vi "SentinelController v35 good v11.vi"() -> ()   [LabVIEW 2011] (continued)
                                n1651 = local read "tester tt start hid"() -> (w1552:u32)
                                n1652 = local read "tester tt end hid"() -> (w1553:u32)
                                n1653 = Subtract(x=w1553, y=w1552) -> (x-y=w1551:u32)
                                n1654 = Divide(x=w1551, y=u32 1000) -> (x/y=w1549:dbl)
                                n1655 = local write "SC measured test time hid"(w1549) -> ()
                                }
                                frame #3 {
                                n1656 = local read "H1 Lock"() -> (w1554:bool)
                                n1657 = case shown="False" w1554 {
                                frame False {
                                n1658 = local read "H2 Lock"() -> (w1555:bool)
                                n1659 = case shown="False" w1555 {
                                frame False {
                                n1660 = One Button Dialog(message="Fatal error 202:\nThe SC responded to a handler being ready with devices\nto test, but when the SC received binning data, no handler had a lock. \nPlease report this bug to Celerint at www.celerint.com  ") -> ()  [unwired: 1 in, 1 out]
                                }
                                frame True {
                                n1661 = local read "H2 online"() -> (w1576:bool)
                                n1662 = local read "Tandem\nfloorspace area"() -> (w1559:i32)
                                n1663 = local read "Std cell \nfloorspace area"() -> (w1587:i32)
                                n1664 = case shown="True" w1576 {
                                tunnel: [0 w1591] -> w1577
                                frame False {
                                }
                                frame True {
                                n1665 = local read "H2 UPH"() -> (w1592:cluster{u32, u32})
                                n1666 = Unbundle(w1592) -> (w1591:u32)  [unwired: 1 out]
                                }
                                }
                                n1667 = local read "System UPH"() -> (w1558:u32)
                                n1668 = local read "UPH"() -> (w1588:dbl)
                                n1669 = Divide(x=w1558, y=w1559) -> (x/y=w1557:dbl)
                                n1670 = local write "Tandem UPH\nper unit area"(w1557) -> ()
                                n1671 = Divide(x=w1588, y=w1587) -> (x/y=w1589:dbl)
                                n1672 = local read "Std hourly\ncost ($/hr)"() -> (w1584:dbl)
                                n1673 = local read "H1 UPH"() -> (w1586:cluster{u32, u32})
                                n1674 = local write "H1 UPH per unit area"(w1589) -> ()
                                n1675 = local read "Utilization (%)"() -> (w1569:u32)
                                n1676 = local read "Tandem hourly\ncost ($/hr)"() -> (w1585:dbl)
                                n1677 = local read "# of devices to test"() -> (w1575:u32)
                                n1678 = Unbundle(w1586) -> (w1578:u32)  [unwired: 1 out]
                                n1679 = local read "Hours per month"() -> (w1570:i32)
                                n1680 = local write "Calc H2 UPH"(w1577) -> ()
                                n1681 = local write "Calc H1 UPH"(w1578) -> ()
                                n1682 = local read "UPH"() -> (w1583:dbl)
                                n1683 = Add(x=w1578, y=w1577) -> (x+y=w1565:u32)
                                n1684 = Divide(x=w1569, y=u32 100) -> (x/y=w1568:dbl)
                                n1685 = Divide(x=w1575, y=w1565) -> (x/y=w1574:dbl)
                                n1686 = Multiply(x=w1570, y=w1568) -> (x*y=w1566:dbl)
                                n1687 = Divide(x=w1584, y=w1583) -> (x/y=w1582:dbl)
                                n1688 = Divide(x=w1585, y=w1565) -> (x/y=w1580:dbl)
                                n1689 = local write "System UPH"(w1565) -> ()
                                n1690 = local write "Calc\nsystem UPH"(w1565) -> ()
                                n1691 = local read "# of devices to test"() -> (w1563:u32)
                                n1692 = Divide(x=w1574, y=w1566) -> (x/y=w1573:dbl)
                                n1693 = Multiply(x=w1582, y=100.0) -> (x*y=w1561:dbl)
                                n1694 = Multiply(x=w1580, y=100.0) -> (x*y=w1560:dbl)
                                n1695 = local write "Std unit cost\n(cents/device)"(w1561) -> ()
                                n1696 = local write "Tandem unit cost\n(cents/device)"(w1560) -> ()
                                n1697 = Subtract(x=w1561, y=w1560) -> (x-y=w1564:dbl)
                                n1698 = Multiply(x=w1573, y=30) -> (x*y=w1571:dbl)
                                n1699 = Multiply(x=w1563, y=w1564) -> (x*y=w1562:dbl)
                                n1700 = local write "Calendar days required\nfor testing all units"(w1571) -> ()
                                n1701 = local write "$ saved"(w1562) -> ()
                                }
                                }
                                }
                                frame True {
                                n1702 = local read "H1 online"() -> (w1613:bool)
                                n1703 = local read "Tandem\nfloorspace area"() -> (w1625:i32)
                                n1704 = local read "Std cell \nfloorspace area"() -> (w1618:i32)
                                n1705 = case shown="True" w1613 {
                                tunnel: [0 w1627] -> w1593
                                frame False {
                                }
                                frame True {
                                n1706 = local read "H1 UPH"() -> (w1628:cluster{u32, u32})
                                n1707 = Unbundle(w1628) -> (w1627:u32)  [unwired: 1 out]
                                }
                                }
                                n1708 = local read "System UPH"() -> (w1624:u32)
                                n1709 = local read "H2 calc UPH"() -> (w1619:dbl)
                                n1710 = Divide(x=w1624, y=w1625) -> (x/y=w1596:dbl)
                                n1711 = Divide(x=w1619, y=w1618) -> (x/y=w1597:dbl)
                                n1712 = local write "Tandem UPH\nper unit area"(w1596) -> ()
                                n1713 = local write "H2 UPH per unit area"(w1597) -> ()
                                n1714 = local read "Std hourly\ncost ($/hr)"() -> (w1621:dbl)
                                n1715 = local read "H2 UPH"() -> (w1623:cluster{u32, u32})
                                n1716 = local read "Utilization (%)"() -> (w1603:u32)
                                n1717 = local read "Tandem hourly\ncost ($/hr)"() -> (w1622:dbl)
                                n1718 = local read "# of devices to test"() -> (w1609:u32)
                                n1719 = local read "Hours per month"() -> (w1604:i32)
                                n1720 = Unbundle(w1623) -> (w1599:u32)  [unwired: 1 out]
                                n1721 = local write "Calc H1 UPH"(w1593) -> ()
                                n1722 = local write "Calc H2 UPH"(w1599) -> ()
                                n1723 = local read "UPH"() -> (w1620:dbl)
                                n1724 = Add(x=w1593, y=w1599) -> (x+y=w1598:u32)
                                n1725 = Divide(x=w1603, y=u32 100) -> (x/y=w1602:dbl)
                                n1726 = local write "System UPH"(w1598) -> ()
                                n1727 = local write "Calc\nsystem UPH"(w1598) -> ()
                                n1728 = Divide(x=w1609, y=w1598) -> (x/y=w1608:dbl)
                                n1729 = Multiply(x=w1604, y=w1602) -> (x*y=w1600:dbl)
                                n1730 = Divide(x=w1621, y=w1620) -> (x/y=w1617:dbl)
                                n1731 = Divide(x=w1622, y=w1598) -> (x/y=w1615:dbl)
                                n1732 = local read "# of devices to test"() -> (w1611:u32)
                                n1733 = Divide(x=w1608, y=w1600) -> (x/y=w1607:dbl)
                                n1734 = Multiply(x=w1617, y=100.0) -> (x*y=w1595:dbl)
                                n1735 = Multiply(x=w1615, y=100.0) -> (x*y=w1594:dbl)
                                n1736 = local write "Std unit cost\n(cents/device)"(w1595) -> ()
                                n1737 = local write "Tandem unit cost\n(cents/device)"(w1594) -> ()
                                n1738 = Subtract(x=w1595, y=w1594) -> (x-y=w1612:dbl)
                                n1739 = Multiply(x=w1607, y=30) -> (x*y=w1605:dbl)
                                n1740 = Multiply(x=w1611, y=w1612) -> (x*y=w1610:dbl)
                                n1741 = local write "Calendar days required\nfor testing all units"(w1605) -> ()
                                n1742 = local write "$ saved"(w1610) -> ()
                                }
                                }
                                }
                                frame #4 {
                                # "when this loop unlocks the handlers,\nthe handler interface loops are free to continue\nto send the binning information to their\nrespective handlers.  Each handler interface \nloop using the \"binning string hidden\" to do\nthis.  That is why, here, there is no writing of\nthe binning informatrion to a handler.  \nThat is done in the handler interface loops."
                                n1743 = local write "H1 Lock"(FALSE ("H1 Lock")) -> ()
                                n1744 = local write "H2 Lock"(FALSE ("H1 Lock")) -> ()
                                }
                                frame #5 {
                                n1745 = local read "Tester online"() -> (w1631:bool)
                                n1746 = local read "POWER"() -> (w1633:bool)
                                n1747 = Compound Arithmetic op=AND(w1631, w1633) -> (w1632:bool)
                                n1748 = case shown="True" w1632 {
                                frame False {
                                n1749 = local write "SC handler states hid"(SC_handler_states."closing bus" ("SC virtual handler states")) -> ()
                                }
                                frame True {
                                n1750 = local write "SC handler states hid"(SC_handler_states."waiting on event" ("SC virtual handler states")) -> ()
                                }
                                }
                                }
                                }
                              }
                              frame "responding to BINON" {
                                n1751 = local read "Last locked handler hid"() -> (w1638:enum16{"H1", "H2"})
                                n1752 = Equal?(x=w1638, y=enum16{"H1", "H2"}."H1") -> (x = y?=w1636:bool)
                                n1753 = case shown="True" w1636 {
                                frame False {
                                n1754 = local read "Last locked handler hid"() -> (w1642:enum16{"H1", "H2"})
                                n1755 = Equal?(x=w1642, y=enum16{"H1", "H2"}."H2") -> (x = y?=w1641:bool)
                                n1756 = case shown="True" w1641 {
                                frame False {
                                }
                                frame True {
                                n1757 = flat-sequence {
                                frame #0 {
                                n1758 = while {
                                stop <- w1646 stop-if-true
                                n1759 = local read "H2 echo hid"() -> (w1644:string)
                                n1760 = String Length(string=w1644) -> (length=w1647:i32)
                                n1761 = Greater Than 0?(x=w1647) -> (x > 0?=w1646:bool)
                                n1762 = Wait (ms)(milliseconds to wait=u32 1) -> ()  [unwired: 1 out]
                                }
                                }
                                frame #1 {
                                # "4"
                                n1763 = local read "GPIB Bus 0 traffic"() -> (w1654:string)
                                n1764 = local read "H2 echo hid"() -> (w1648:string)
                                n1765 = local read "VISA bus 0 resource name out hid"() -> (w1658:refnum<visa-resource-name>)
                                n1766 = local read "VISA bus 0 error out hid"() -> (w1657:errorcluster)
                                n1767 = call <vilib>:"Trim Whitespace.vi"("string"=w1648) -> ("trimmed string"=w1649:string)  [unwired: 1 in]
                                n1768 = VISA Write(VISA resource name=w1658, write buffer=w1648, error in (no error)=w1657) -> (VISA resource name out=w1656:refnum<visa-resource-name>, error out=w1655:errorcluster)  [unwired: 1 out]
                                n1769 = Concatenate Strings(w1654, "\r\n", "Bus 0 write: " ("string"), w1649) -> (w1652:string)
                                n1770 = local write "VISA bus 0 resource name out hid"(w1656) -> ()
                                n1771 = Unbundle By Name(w1655) -> ("status"=w1650:bool)
                                n1772 = local write "VISA bus 0 error out hid"(w1655) -> ()
                                n1773 = local write "GPIB Bus 0 traffic"(w1652) -> ()
                                n1774 = local write "GPIB bus 0 write error"(w1650) -> ()
                                }
                                frame #2 {
                                n1775 = local write "SC handler states hid"(SC_handler_states."waiting on event" ("SC Test Interface States")) -> ()
                                }
                                }
                                }
                                }
                                }
                                frame True {
                                n1776 = flat-sequence {
                                frame #0 {
                                n1777 = while {
                                i -> [w1660]
                                stop <- w1662 stop-if-true
                                n1778 = local read "H1 echo hid"() -> (w1664:string)
                                n1779 = String Length(string=w1664) -> (length=w1663:i32)
                                n1780 = Greater Than 0?(x=w1663) -> (x > 0?=w1662:bool)
                                n1781 = Wait (ms)(milliseconds to wait=u32 1) -> ()  [unwired: 1 out]
                                "Numeric 4" <- w1660
                                }
                                }
                                frame #1 {
                                n1782 = local read "GPIB Bus 0 traffic"() -> (w1671:string)
                                n1783 = local read "VISA bus 0 resource name out hid"() -> (w1675:refnum<visa-resource-name>)
                                n1784 = local read "H1 echo hid"() -> (w1665:string)
                                n1785 = local read "VISA bus 0 error out hid"() -> (w1674:errorcluster)
                                n1786 = VISA Write(VISA resource name=w1675, write buffer=w1665, error in (no error)=w1674) -> (VISA resource name out=w1673:refnum<visa-resource-name>, error out=w1672:errorcluster)  [unwired: 1 out]
                                n1787 = call <vilib>:"Trim Whitespace.vi"("string"=w1665) -> ("trimmed string"=w1666:string)  [unwired: 1 in]
                                n1788 = local write "VISA bus 0 resource name out hid"(w1673) -> ()
                                n1789 = Unbundle By Name(w1672) -> ("status"=w1667:bool)
                                n1790 = local write "VISA bus 0 error out hid"(w1672) -> ()
                                n1791 = Concatenate Strings(w1671, "\r\n", "Bus 0 write: " ("string"), w1666) -> (w1669:string)
                                n1792 = local write "GPIB bus 0 write error"(w1667) -> ()
                                n1793 = local write "GPIB Bus 0 traffic"(w1669) -> ()
                                }
                                frame #2 {
                                n1794 = local write "SC handler states hid"(SC_handler_states."waiting on event" ("SC Test Interface States")) -> ()
                                }
                                }
                                }
                                }
                              }
                              frame "ECHONG" {
                                n1795 = flat-sequence {
                                frame #0 {
                                # "Echo was returned to the tester via the BINON state"
                                n1796 = local read "H1 Lock"() -> (w1679:bool)
                                n1797 = case shown="True" w1679 {
                                frame False {
                                n1798 = local read "H2 Lock"() -> (w1680:bool)
                                n1799 = case shown="True" w1680 {
                                frame False {
                                }
                                frame True {
                                n1800 = local read "GPIB Bus 0 traffic"() -> (w1684:string)
                                n1801 = Concatenate Strings(w1684, "\r\n", "Bus 0: ECHONG received for H2. Retrying." ("string")) -> (w1682:string)
                                n1802 = local write "GPIB Bus 0 traffic"(w1682) -> ()
                                }
                                }
                                }
                                frame True {
                                n1803 = local read "GPIB Bus 0 traffic"() -> (w1688:string)
                                n1804 = Concatenate Strings(w1688, "\r\n", "Bus 0: ECHONG received for H1. Retrying." ("string")) -> (w1686:string)
                                n1805 = local write "GPIB Bus 0 traffic"(w1686) -> ()
                                }
                                }
                                }
                                frame #1 {
                                n1806 = local write "SC handler states hid"(SC_handler_states."waiting on event" ("SC Test Interface States")) -> ()
                                }
                                }
                              }
                              frame "ECHOOK" {
                                n1807 = flat-sequence {
                                frame #0 {
                                # "Echo was returned to the tester via the BINON state"
                                n1808 = local read "Last locked handler hid"() -> (w1694:enum16{"H1", "H2"})
                                n1809 = Equal?(x=w1694, y=enum16{"H1", "H2"}."H1") -> (x = y?=w1692:bool)
                                n1810 = case shown="True" w1692 {
                                frame False {
                                n1811 = local read "Last locked handler hid"() -> (w1696:enum16{"H1", "H2"})
                                n1812 = Equal?(x=w1696, y=enum16{"H1", "H2"}."H2") -> (x = y?=w1695:bool)
                                n1813 = case shown="True" w1695 {
                                frame False {
                                }
                                frame True {
                                n1814 = local read "GPIB Bus 0 traffic"() -> (w1701:string)
                                n1815 = Concatenate Strings(w1701, "\r\n", "Bus 0: ECHOOK received for H2." ("string")) -> (w1699:string)
                                n1816 = local write "GPIB Bus 0 traffic"(w1699) -> ()
                                }
                                }
                                }
                                frame True {
                                n1817 = local read "GPIB Bus 0 traffic"() -> (w1705:string)
                                n1818 = Concatenate Strings(w1705, "\r\n", "Bus 0: ECHOOK received for H1." ("string")) -> (w1703:string)
                                n1819 = local write "GPIB Bus 0 traffic"(w1703) -> ()
                                }
                                }
                                }
                                frame #1 {
                                n1820 = Tick Count (ms)() -> (millisecond timer value=w1706:u32)
                                n1821 = Tick Count (ms)() -> (millisecond timer value=w1707:u32)
                                n1822 = local write "tester wt start hid"(w1706) -> ()
                                n1823 = local write "tester tt end hid"(w1707) -> ()
                                }
                                frame #2 {
                                n1824 = local read "tester tt start hid"() -> (w1711:u32)
                                n1825 = local read "tester tt end hid"() -> (w1712:u32)
                                n1826 = Subtract(x=w1712, y=w1711) -> (x-y=w1710:u32)
                                n1827 = Divide(x=w1710, y=u32 1000) -> (x/y=w1708:dbl)
                                n1828 = local write "SC measured test time hid"(w1708) -> ()
                                }
                                frame #3 {
                                n1829 = local read "Last locked handler hid"() -> (w1713:enum16{"H1", "H2"})
                                n1830 = case shown="\"H1\", Default" w1713 {
                                frame "H1", Default {
                                n1831 = local read "H1 online"() -> (w1734:bool)
                                n1832 = local read "Tandem\nfloorspace area"() -> (w1746:i32)
                                n1833 = local read "Std cell \nfloorspace area"() -> (w1739:i32)
                                n1834 = case shown="True" w1734 {
                                tunnel: [0 w1748] -> w1714
                                frame False {
                                }
                                frame True {
                                n1835 = local read "H1 UPH"() -> (w1749:cluster{u32, u32})
                                n1836 = Unbundle(w1749) -> (w1748:u32)  [unwired: 1 out]
                                }
                                }
                                n1837 = local read "System UPH"() -> (w1745:u32)
                                n1838 = local read "H2 calc UPH"() -> (w1740:dbl)
                                n1839 = Divide(x=w1745, y=w1746) -> (x/y=w1717:dbl)
                                n1840 = Divide(x=w1740, y=w1739) -> (x/y=w1718:dbl)
                                n1841 = local write "Tandem UPH\nper unit area"(w1717) -> ()
                                n1842 = local write "H2 UPH per unit area"(w1718) -> ()
                                n1843 = local read "Std hourly\ncost ($/hr)"() -> (w1742:dbl)
                                n1844 = local read "H2 UPH"() -> (w1744:cluster{u32, u32})
                                n1845 = local read "Utilization (%)"() -> (w1724:u32)
                                n1846 = local read "Tandem hourly\ncost ($/hr)"() -> (w1743:dbl)
                                n1847 = local read "# of devices to test"() -> (w1730:u32)
                                n1848 = local read "Hours per month"() -> (w1725:i32)
                                n1849 = Unbundle(w1744) -> (w1720:u32)  [unwired: 1 out]
                                n1850 = local write "Calc H1 UPH"(w1714) -> ()
                                n1851 = local write "Calc H2 UPH"(w1720) -> ()
                                n1852 = local read "UPH"() -> (w1741:dbl)
                                n1853 = Add(x=w1714, y=w1720) -> (x+y=w1719:u32)
                                n1854 = Divide(x=w1724, y=u32 100) -> (x/y=w1723:dbl)
                                n1855 = Divide(x=w1742, y=w1741) -> (x/y=w1738:dbl)
                                n1856 = Divide(x=w1743, y=w1719) -> (x/y=w1736:dbl)
                                n1857 = Divide(x=w1730, y=w1719) -> (x/y=w1729:dbl)
                                n1858 = Multiply(x=w1725, y=w1723) -> (x*y=w1721:dbl)
                                n1859 = local write "System UPH"(w1719) -> ()
                                n1860 = local write "Calc\nsystem UPH"(w1719) -> ()
                                n1861 = local read "# of devices to test"() -> (w1732:u32)
                                n1862 = Divide(x=w1729, y=w1721) -> (x/y=w1728:dbl)
                                n1863 = Multiply(x=w1738, y=100.0) -> (x*y=w1716:dbl)
                                n1864 = Multiply(x=w1736, y=100.0) -> (x*y=w1715:dbl)
                                n1865 = local write "Tandem unit cost\n(cents/device)"(w1715) -> ()
                                n1866 = local write "Std unit cost\n(cents/device)"(w1716) -> ()
                                n1867 = Subtract(x=w1716, y=w1715) -> (x-y=w1733:dbl)
                                n1868 = Multiply(x=w1728, y=30) -> (x*y=w1726:dbl)
                                n1869 = Multiply(x=w1732, y=w1733) -> (x*y=w1731:dbl)
                                n1870 = local write "Calendar days required\nfor testing all units"(w1726) -> ()
                                n1871 = local write "$ saved"(w1731) -> ()
                                }
                                frame "H2" {
                                n1872 = local read "H2 online"() -> (w1769:bool)
                                n1873 = local read "Tandem\nfloorspace area"() -> (w1752:i32)
                                n1874 = local read "Std cell \nfloorspace area"() -> (w1780:i32)
                                n1875 = case shown="True" w1769 {
                                tunnel: [0 w1784] -> w1770
                                frame False {
                                }
                                frame True {
                                n1876 = local read "H2 UPH"() -> (w1785:cluster{u32, u32})
                                n1877 = Unbundle(w1785) -> (w1784:u32)  [unwired: 1 out]
                                }
                                }
                                n1878 = local read "System UPH"() -> (w1751:u32)
                                n1879 = local read "UPH"() -> (w1781:dbl)
                                n1880 = Divide(x=w1751, y=w1752) -> (x/y=w1750:dbl)
                                n1881 = local write "Tandem UPH\nper unit area"(w1750) -> ()
                                n1882 = Divide(x=w1781, y=w1780) -> (x/y=w1782:dbl)
                                n1883 = local read "Std hourly\ncost ($/hr)"() -> (w1777:dbl)
                                n1884 = local read "H1 UPH"() -> (w1779:cluster{u32, u32})
                                n1885 = local read "Utilization (%)"() -> (w1762:u32)
                                n1886 = local write "H1 UPH per unit area"(w1782) -> ()
                                n1887 = local read "Tandem hourly\ncost ($/hr)"() -> (w1778:dbl)
                                n1888 = local read "# of devices to test"() -> (w1768:u32)
                                n1889 = Unbundle(w1779) -> (w1771:u32)  [unwired: 1 out]
                                n1890 = local read "Hours per month"() -> (w1763:i32)
                                n1891 = local write "Calc H1 UPH"(w1771) -> ()
                                n1892 = local write "Calc H2 UPH"(w1770) -> ()
                                n1893 = local read "UPH"() -> (w1776:dbl)
                                n1894 = Add(x=w1771, y=w1770) -> (x+y=w1758:u32)
                                n1895 = Divide(x=w1762, y=u32 100) -> (x/y=w1761:dbl)
                                n1896 = Divide(x=w1777, y=w1776) -> (x/y=w1775:dbl)
                                n1897 = Divide(x=w1778, y=w1758) -> (x/y=w1773:dbl)
                                n1898 = Divide(x=w1768, y=w1758) -> (x/y=w1767:dbl)
                                n1899 = Multiply(x=w1763, y=w1761) -> (x*y=w1759:dbl)
                                n1900 = local write "System UPH"(w1758) -> ()
                                n1901 = local write "Calc\nsystem UPH"(w1758) -> ()
                                n1902 = local read "# of devices to test"() -> (w1756:u32)
                                n1903 = Divide(x=w1767, y=w1759) -> (x/y=w1766:dbl)
                                n1904 = Multiply(x=w1775, y=100.0) -> (x*y=w1754:dbl)
                                n1905 = Multiply(x=w1773, y=100.0) -> (x*y=w1753:dbl)
                                n1906 = local write "Tandem unit cost\n(cents/device)"(w1753) -> ()
                                n1907 = local write "Std unit cost\n(cents/device)"(w1754) -> ()
                                n1908 = Subtract(x=w1754, y=w1753) -> (x-y=w1757:dbl)
                                n1909 = Multiply(x=w1766, y=30) -> (x*y=w1764:dbl)
                                n1910 = Multiply(x=w1756, y=w1757) -> (x*y=w1755:dbl)
                                n1911 = local write "Calendar days required\nfor testing all units"(w1764) -> ()
                                n1912 = local write "$ saved"(w1755) -> ()
                                }
                                }
                                }
                                frame #4 {
                                n1913 = local read "Tester online"() -> (w1786:bool)
                                n1914 = local read "POWER"() -> (w1788:bool)
                                n1915 = Compound Arithmetic op=AND(w1786, w1788) -> (w1787:bool)
                                n1916 = case shown="True" w1787 {
                                frame False {
                                n1917 = local write "SC handler states hid"(SC_handler_states."closing bus" ("SC virtual handler states")) -> ()
                                }
                                frame True {
                                n1918 = local write "SC handler states hid"(SC_handler_states."waiting on serial poll" ("SC Test Interface States")) -> ()
                                }
                                }
                                }
                                }
                              }
                              frame "closing bus" {
                                n1919 = flat-sequence {
                                frame #0 {
                                n1920 = local read "GPIB Bus 0 traffic"() -> (w1796:string)
                                n1921 = Concatenate Strings(w1796, "\r\n", "Bus 0 closing: " ("string")) -> (w1794:string)
                                n1922 = local write "GPIB Bus 0 traffic"(w1794) -> ()
                                }
                                frame #1 {
                                n1923 = local read "VISA bus 0 resource name out hid"() -> (w1798:refnum<visa-resource-name>)
                                n1924 = local read "VISA bus 0 error out hid"() -> (w1799:errorcluster)
                                n1925 = VISA Close(VISA resource name=w1798, error in (no error)=w1799) -> (error out=w1797:errorcluster)
                                n1926 = Unbundle By Name(w1797) -> ("status"=w1800:bool)
                                n1927 = local write "VISA bus 0 close error"(w1800) -> ()
                                }
                                frame #2 {
                                n1928 = local write "Exit SC handler StMach hid"(TRUE ("Exit tester state machine hid")) -> ()
                                }
                                }
                              }
                              frame "responding to unknown command" {
                                n1929 = flat-sequence {
                                frame #0 {
                                n1930 = local read "GPIB Bus 0 traffic"() -> (w1808:string)
                                n1931 = Concatenate Strings(w1808, "\r\n", "Bus 0 write: " ("string"), "unrecognized string") -> (w1806:string)
                                n1932 = local write "GPIB Bus 0 traffic"(w1806) -> ()
                                }
                                frame #1 {
                                n1933 = local write "SC handler states hid"(SC_handler_states."waiting on event" ("SC Test Interface States")) -> ()
                                }
                                }
                              }
                            }
                          }
                          frame #1 {
                            n1934 = local read "Slow for  Diagnostics"() -> (w1810:bool)
                            n1935 = case shown="True" w1810 {
                              frame False {
                              }
                              frame True {
                                n1936 = local read "GPIB wait time (ms)"() -> (w1813:u32)
                                n1937 = Wait (ms)(milliseconds to wait=w1813) -> ()  [unwired: 1 out]
                              }
                            }
                          }
                        }
                        n1938 = Wait (ms)(milliseconds to wait=u32 1) -> ()  [unwired: 1 out]
                        n1939 = local read "Exit SC handler StMach hid"() -> (w1076:bool)
                        "Numeric" <- w1072
                      }
                    }
                  }
                }
              }
              n1940 = Wait (ms)(milliseconds to wait=u32 5) -> ()  [unwired: 1 out]
              n1941 = local read "POWER"() -> (w1062:bool)
            }
            n1942 = while {
              stop <- w360 continue-if-true
              n1943 = local read "H1 online"() -> (w361:bool)
              n1944 = case shown="True" w361 {
                frame False {
                }
                frame True {
                  n1945 = flat-sequence {
                    frame #0 {
                      n1946 = local write "Exit SC tester H1 StMach hid"(FALSE ("Exit H1 state machine hid")) -> ()
                    }
                    frame #1 {
                      n1947 = local read "H1 handler type"() -> (w363:T2)
                      n1948 = case shown="\"Seiko-Epson NS6040\"" w363 {
                        frame "Multitest", Default {
                          n1949 = local write "MT99XX tester states H1 hid"(SC_MT99XX_tester_states."initializing bus" ("SC virtual tester states")) -> ()
                          n1950 = flat-sequence {
                            frame #0 {
                              n1951 = local read "MT99XX tester states H1 hid"() -> (w365:T5)
                              n1952 = case shown="\"polling *SITES?\"" w365 {
                                frame "initializing bus", Default {
                                n1953 = flat-sequence {
                                frame #0 {
                                # "bus 1"
                                n1954 = local read "GPIB wait timeout hid"() -> (w369:u32)
                                n1955 = local read "SentCtrl talks to handler 1 at"() -> (w370:refnum<visa-resource-name>)
                                n1956 = local read "GPIB wait timeout hid"() -> (w368:u32)
                                n1957 = VISA Open(timeout (0)=w369, VISA resource name=w370) -> (VISA resource name=w367:refnum<visa-resource-name>, error out=w372:errorcluster)  [unwired: 3 in]
                                n1958 = property class="GPIB Instr"(reference=w367, error in=w372, "Timeout"=w368) -> (error out=w366:errorcluster)  [unwired: 1 out]
                                n1959 = local write "VISA bus 1 resource name out hid"(w367) -> ()
                                n1960 = Unbundle By Name(w366) -> ("status"=w371:bool)
                                n1961 = local write "VISA bus 1 open error"(w371) -> ()
                                n1962 = local write "VISA bus 1 error out hid"(w366) -> ()
                                }
                                frame #1 {
                                n1963 = local write "Exit SC tester H1 StMach hid"(FALSE ("Exit H1 state machine hid")) -> ()
                                n1964 = Concatenate Strings("Bus 1 initializing" ("string"), "\r\n") -> (w375:string)
                                n1965 = local write "GPIB bus 1 traffic"(w375) -> ()
                                }
                                frame #2 {
                                n1966 = local write "MT99XX tester states H1 hid"(SC_MT99XX_tester_states."sending *IDN?" ("SC virtual tester states")) -> ()
                                }
                                }
                                }
                                frame "sending *IDN?" {
                                n1967 = flat-sequence {
                                tunnel: [w387] -> w380
                                tunnel: [w386] -> w379
                                tunnel: w380 -> [w401]
                                tunnel: w379 -> [w400]
                                tunnel: [w391] -> w378
                                tunnel: w378 -> [w402]
                                frame #0 {
                                w381 = "*IDN?"
                                n1968 = local read "VISA bus 1 resource name out hid"() -> (w390:refnum<visa-resource-name>)
                                n1969 = local read "GPIB bus 1 traffic"() -> (w385:string)
                                n1970 = local read "VISA bus 1 error out hid"() -> (w389:errorcluster)
                                n1971 = Concatenate Strings(w385, "\r\n", "Bus 1 write: " ("string"), w381) -> (w383:string)
                                n1972 = VISA Write(VISA resource name=w390, write buffer=w381, error in (no error)=w389) -> (VISA resource name out=w387:refnum<visa-resource-name>, error out=w386:errorcluster)  [unwired: 1 out]
                                n1973 = Unbundle By Name(w386) -> ("status"=w388:bool)
                                n1974 = local write "GPIB bus 1 traffic"(w383) -> ()
                                n1975 = local write "GPIB bus 1 write error"(w388) -> ()
                                }
                                frame #1 {
                                n1976 = local read "GPIB bus 1 traffic"() -> (w393:string)
                                n1977 = VISA Read(VISA resource name=w401, byte count=u32 256, error in (no error)=w400) -> (VISA resource name out=w398:refnum<visa-resource-name>, read buffer=w392:string, error out=w397:errorcluster)  [unwired: 1 out]
                                n1978 = local write "VISA bus 1 resource name out hid"(w398) -> ()
                                n1979 = Unbundle By Name(w397) -> ("status"=w391:bool)
                                n1980 = local write "H1 response to *IDN? hid"(w392) -> ()
                                n1981 = local write "GPIB bus 1 read error"(w391) -> ()
                                n1982 = Concatenate Strings(w393, "\r\n", "Bus 1 read: " ("string"), w392) -> (w395:string)
                                n1983 = local write "GPIB bus 1 traffic"(w395) -> ()
                                }
                                frame #2 {
                                n1984 = case shown="False" w402 {
                                frame False {
                                n1985 = local write "MT99XX tester states H1 hid"(SC_MT99XX_tester_states."polling *SITES?" ("SC virtual tester states")) -> ()
                                }
                                frame True {
                                n1986 = flat-sequence {
                                frame #0 {
                                n1987 = while {
                                stop <- w405 stop-if-true
                                n1988 = One Button Dialog(message="Warning:\nVirtual tester does not get a response\nto *IDN? from handler 1.\nCheck GPIB cable and that  handler 1 \nis running and ready to issue a start of test\nby responding with sites ready.", button name ("OK")="Dismiss and retry") -> (true=w405:bool)
                                n1989 = Wait (ms)(milliseconds to wait=u32 100) -> ()  [unwired: 1 out]
                                }
                                }
                                frame #1 {
                                n1990 = local write "H1 online"(FALSE ("H1 online")) -> ()
                                }
                                frame #2 {
                                n1991 = local write "MT99XX tester states H1 hid"(SC_MT99XX_tester_states."sending *IDN?" ("SC virtual tester states")) -> ()
                                }
                                }
                                }
                                }
                                }
                                }
                                }
                                frame "polling *SITES?" {
                                n1992 = flat-sequence {
                                tunnel: [w413] -> w411
                                tunnel: [w412] -> w410
                                tunnel: w411 -> [w449]
                                tunnel: w410 -> [w448]
                                frame #0 {
                                n1993 = while {
                                tunnel: [w417] -> w413
                                tunnel: [w415] -> w412
                                stop <- w414 stop-if-true
                                n1994 = stacked-sequence {
                                tunnel: [w429] -> w419
                                tunnel: [w428] -> w418
                                frame #0 {
                                w421 = "*SITES?"
                                n1995 = local read "VISA bus 1 resource name out hid"() -> (w427:refnum<visa-resource-name>)
                                n1996 = local read "VISA bus 1 error out hid"() -> (w426:errorcluster)
                                n1997 = Concatenate Strings("Handler 1 cycle start" ("string"), "\r\n", "Bus 1 write: " ("string"), w421) -> (w423:string)
                                n1998 = VISA Write(VISA resource name=w427, write buffer=w421, error in (no error)=w426) -> (VISA resource name out=w429:refnum<visa-resource-name>, error out=w428:errorcluster)  [unwired: 1 out]
                                n1999 = Unbundle By Name(w428) -> ("status"=w425:bool)
                                n2000 = local write "GPIB bus 1 traffic"(w423) -> ()
                                n2001 = local write "GPIB bus 1 write error"(w425) -> ()
                                }
                                }
                                n2002 = Wait (ms)(milliseconds to wait=u32 1) -> ()  [unwired: 1 out]
                                n2003 = flat-sequence {
                                tunnel: w419 -> [w447]
                                tunnel: w418 -> [w446]
                                tunnel: [w434] -> w417
                                tunnel: [w430] -> w415
                                tunnel: [w431] -> w414
                                frame #0 {
                                n2004 = local read "GPIB bus 1 traffic"() -> (w439:string)
                                n2005 = VISA Read(VISA resource name=w447, byte count=u32 256, error in (no error)=w446) -> (read buffer=w434:string, error out=w433:errorcluster)  [unwired: 2 out]
                                n2006 = Unbundle By Name(w433) -> ("status"=w430:bool)
                                n2007 = String Length(string=w434) -> (length=w436:i32)
                                n2008 = Scan Value(string=w434, format string="%b", default (0 dbl)=u8 0) -> (value=w438:u8)  [unwired: 1 out]
                                n2009 = Concatenate Strings(w439, "\r\n", "Bus 1 read: " ("string"), w434) -> (w441:string)
                                n2010 = local write "GPIB bus 1 read error"(w430) -> ()
                                n2011 = Greater Than 0?(x=w436) -> (x > 0?=w435:bool)
                                n2012 = Greater Than 0?(x=w438) -> (x > 0?=w437:bool)
                                n2013 = local write "GPIB bus 1 traffic"(w441) -> ()
                                n2014 = And(x=w435, y=w437) -> (x .and. y?=w432:bool)
                                n2015 = Or(x=w432, y=w430) -> (x .or. y?=w431:bool)
                                }
                                }
                                }
                                }
                                frame #1 {
                                n2016 = case shown="False" w448 {
                                tunnel: w449 -> [w450 _]
                                frame False {
                                n2017 = flat-sequence {
                                tunnel: w450 -> [w451]
                                frame #0 {
                                n2018 = String Length(string=w451) -> (length=w452:i32)
                                n2019 = local write "H1 SITES? response hid"(w451) -> ()
                                n2020 = local write "H1 parallelism"(w452) -> ()
                                }
                                frame #1 {
                                # "This block adds zeroes (sites not ready)\nto SITES READY from handlers when the\nhandler is running at a lower parallelism\nthan the test program, but has the same\npin mapping for the active sites in common."
                                n2021 = local read "Program Parallelism"() -> (w456:u32)
                                n2022 = local read "H1 allow lower parallelism"() -> (w455:bool)
                                n2023 = local read "H1 parallelism"() -> (w457:u32)
                                n2024 = Less?(x=w457, y=w456) -> (x < y?=w454:bool)
                                n2025 = And(x=w454, y=w455) -> (x .and. y?=w453:bool)
                                n2026 = case shown="True" w453 {
                                frame False {
                                n2027 = local read "Program Parallelism"() -> (w460:u32)
                                n2028 = local read "H1 parallelism"() -> (w458:u32)
                                n2029 = Greater?(x=w458, y=w460) -> (0:w459:bool)
                                n2030 = case shown="True" w459 {
                                frame False {
                                # "parallelisms must match if arriving here"
                                n2031 = local write "MT99XX tester states H1 hid"(SC_MT99XX_tester_states."testing" ("SC virtual tester states")) -> ()
                                }
                                frame True {
                                n2032 = local write "MT99XX tester states H1 hid"(SC_MT99XX_tester_states."closing bus" ("SC virtual tester states")) -> ()
                                n2033 = local write "POWER"(FALSE ("POWER")) -> ()
                                n2034 = One Button Dialog(message="Fatal error 300:\nTest program cannot support higher\nparallelism on handler 1.\nThe Sentinel Controller program is shutting down.\nPlease correct the mismatch and restart.") -> ()  [unwired: 1 in, 1 out]
                                }
                                }
                                }
                                frame True {
                                n2035 = local read "Program Parallelism"() -> (w470:u32)
                                n2036 = local read "H1 parallelism"() -> (w467:u32)
                                n2037 = local read "H1 SITES? response hid"() -> (w468:string)
                                n2038 = Subtract(x=w470, y=w467) -> (x-y=w469:u32)
                                n2039 = for {
                                N: w469 -> [_]
                                shift-right: [w471] -> w465
                                shift-left: w468 -> [w472]
                                n2040 = Concatenate Strings(w472, "0" ("string")) -> (w471:string)
                                }
                                n2041 = local write "H1 SITES? response hid"(w465) -> ()
                                n2042 = local write "MT99XX tester states H1 hid"(SC_MT99XX_tester_states."testing" ("SC virtual tester states")) -> ()
                                }
                                }
                                }
                                frame #2 {
                                n2043 = Tick Count (ms)() -> (millisecond timer value=w478:u32)
                                n2044 = Tick Count (ms)() -> (millisecond timer value=w477:u32)
                                n2045 = local write "H1 Ready with sites"(TRUE ("H2 Waiting")) -> ()
                                n2046 = local write "H1 wt start hidden"(w478) -> ()
                                n2047 = local write "H1 it end hidden"(w477) -> ()
                                n2048 = local write "H1 Indexing"(FALSE ("h1 indexing")) -> ()
                                n2049 = local write "H1 Testing"(FALSE ("h1 indexing")) -> ()
                                }
                                frame #3 {
                                n2050 = local read "H1 it start hidden"() -> (w482:u32)
                                n2051 = local read "H1 it end hidden"() -> (w483:u32)
                                n2052 = Subtract(x=w483, y=w482) -> (x-y=w479:u32)
                                n2053 = Divide(x=w479, y=u32 1000) -> (x/y=w481:dbl)
                                n2054 = local write "MT99XX tester states H1 hid"(SC_MT99XX_tester_states."testing" ("SC virtual tester states")) -> ()
                                n2055 = local write "H1 measured Index Time"(w481) -> ()
                                }
                                }
                                }
                                frame True {
                                n2056 = flat-sequence {
                                frame #0 {
                                n2057 = local read "VISA bus 1 resource name out hid"() -> (w487:refnum<visa-resource-name>)
                                n2058 = local read "VISA bus 1 error out hid"() -> (w488:errorcluster)
                                n2059 = VISA Close(VISA resource name=w487, error in (no error)=w488) -> (error out=w486:errorcluster)
                                n2060 = Unbundle By Name(w486) -> ("status"=w485:bool)
                                n2061 = local write "VISA bus 1 close error"(w485) -> ()
                                }
                                frame #1 {
                                n2062 = local write "VISA bus 1 close error"(FALSE ("VISA bus 1 close error")) -> ()
                                n2063 = Concatenate Strings("Bus 1 error  while reading,\nclosing Bus 1 and re-initializing" ("string"), "\r\n") -> (w491:string)
                                n2064 = local write "GPIB bus 1 traffic"(w491) -> ()
                                }
                                frame #2 {
                                n2065 = local write "MT99XX tester states H1 hid"(SC_MT99XX_tester_states."initializing bus" ("SC virtual tester states")) -> ()
                                }
                                }
                                }
                                }
                                }
                                }
                                }
                                frame "testing" {
                                n2066 = flat-sequence {
                                frame #0 {
                                n2067 = while {
                                stop <- w494 stop-if-true
                                n2068 = local read "H1 Lock"() -> (w494:bool)
                                n2069 = Wait (ms)(milliseconds to wait=u32 1) -> ()  [unwired: 1 out]
                                }
                                }
                                frame #1 {
                                n2070 = Tick Count (ms)() -> (millisecond timer value=w505:u32)
                                n2071 = Tick Count (ms)() -> (millisecond timer value=w504:u32)
                                n2072 = local write "H1 Testing"(TRUE ("testing")) -> ()
                                n2073 = local write "H1 Ready with sites"(FALSE ("H1 Waiting")) -> ()
                                n2074 = local write "H1 Indexing"(FALSE ("waiting")) -> ()
                                n2075 = local write "H1 wt end hidden"(w505) -> ()
                                n2076 = local write "H1 tt start hidden"(w504) -> ()
                                n2077 = local read "GPIB bus 1 traffic"() -> (w497:string)
                                n2078 = Concatenate Strings(w497, "\r\n", "Bus 1: " ("string"), "testing" ("string")) -> (w499:string)
                                n2079 = local write "GPIB bus 1 traffic"(w499) -> ()
                                }
                                frame #2 {
                                n2080 = local read "H1 wt start hidden"() -> (w509:u32)
                                n2081 = local read "H1 wt end hidden"() -> (w510:u32)
                                n2082 = Subtract(x=w510, y=w509) -> (x-y=w508:u32)
                                n2083 = Divide(x=w508, y=u32 1000) -> (x/y=w506:dbl)
                                n2084 = local write "H1 measured Wait Time"(w506) -> ()
                                }
                                frame #3 {
                                n2085 = local write "MT99XX tester states H1 hid"(SC_MT99XX_tester_states."binning" ("SC virtual tester states")) -> ()
                                }
                                }
                                }
                                frame "binning" {
                                n2086 = flat-sequence {
                                tunnel: [w523] -> w514
                                tunnel: [w550] -> w515
                                tunnel: w514 -> [w550]
                                tunnel: w515 -> [w557]
                                tunnel: [w556] -> w513
                                tunnel: [w555] -> w512
                                tunnel: w513 -> [w608]
                                tunnel: w512 -> [w607]
                                frame #0 {
                                n2087 = while {
                                stop <- w517 continue-if-true
                                n2088 = local read "H1 Lock"() -> (w517:bool)
                                n2089 = Wait (ms)(milliseconds to wait=u32 1) -> ()  [unwired: 1 out]
                                }
                                }
                                frame #1 {
                                n2090 = local read "Program Parallelism"() -> (w521:u32)
                                n2091 = local read "H1 parallelism"() -> (w522:u32)
                                n2092 = Less?(x=w522, y=w521) -> (x < y?=w519:bool)
                                n2093 = local read "H1 allow lower parallelism"() -> (w520:bool)
                                n2094 = And(x=w519, y=w520) -> (x .and. y?=w518:bool)
                                n2095 = case shown="False" w518 {
                                tunnel: [w524 w535] -> w523
                                frame False {
                                n2096 = local read "VISA bus 1 resource name out hid"() -> (w532:refnum<visa-resource-name>)
                                n2097 = local read "Binning string from tester hid"() -> (w524:string)
                                n2098 = local read "VISA bus 1 error out hid"() -> (w533:errorcluster)
                                n2099 = local read "GPIB bus 1 traffic"() -> (w528:string)
                                n2100 = VISA Write(VISA resource name=w532, write buffer=w524, error in (no error)=w533) -> (VISA resource name out=w530:refnum<visa-resource-name>, error out=w531:errorcluster)  [unwired: 1 out]
                                n2101 = local write "VISA bus 1 resource name out hid"(w530) -> ()
                                n2102 = local write "VISA bus 1 error out hid"(w531) -> ()
                                n2103 = Unbundle By Name(w531) -> ("status"=w529:bool)
                                n2104 = Concatenate Strings(w528, "\r\n", "Bus 1 write: " ("string"), w524) -> (w526:string)
                                n2105 = local write "GPIB bus 1 write error"(w529) -> ()
                                n2106 = local write "GPIB bus 1 traffic"(w526) -> ()
                                }
                                frame True {
                                n2107 = local read "H1 parallelism"() -> (w534:u32)
                                n2108 = local read "Binning string from tester hid"() -> (w536:string)
                                n2109 = local read "VISA bus 1 resource name out hid"() -> (w547:refnum<visa-resource-name>)
                                n2110 = local read "VISA bus 1 error out hid"() -> (w548:errorcluster)
                                n2111 = Multiply(x=w534, y=u32 8) -> (x*y=w538:u32)
                                n2112 = local read "GPIB bus 1 traffic"() -> (w543:string)
                                n2113 = Decrement(x=w538) -> (x-1=w539:u32)
                                n2114 = String Subset(string=w536, length (rest)=w539) -> (substring=w535:string)  [unwired: 1 in]
                                n2115 = VISA Write(VISA resource name=w547, write buffer=w535, error in (no error)=w548) -> (VISA resource name out=w545:refnum<visa-resource-name>, error out=w546:errorcluster)  [unwired: 1 out]
                                n2116 = local write "VISA bus 1 resource name out hid"(w545) -> ()
                                n2117 = local write "VISA bus 1 error out hid"(w546) -> ()
                                n2118 = Unbundle By Name(w546) -> ("status"=w544:bool)
                                n2119 = Concatenate Strings(w543, "\r\n", "Bus 1 write: " ("string"), w535) -> (w541:string)
                                n2120 = local write "GPIB bus 1 traffic"(w541) -> ()
                                n2121 = local write "GPIB bus 1 write error"(w544) -> ()
                                }
                                }
                                }
                                frame #2 {
                                n2122 = local write "H1 Ready with sites"(FALSE ("waiting")) -> ()
                                n2123 = Tick Count (ms)() -> (millisecond timer value=w551:u32)
                                n2124 = Tick Count (ms)() -> (millisecond timer value=w552:u32)
                                n2125 = local write "H1 tt end hidden"(w551) -> ()
                                n2126 = local write "H1 it start hidden"(w552) -> ()
                                n2127 = local write "H1 Indexing"(TRUE ("waiting")) -> ()
                                n2128 = local write "H1 Testing"(FALSE ("waiting")) -> ()
                                }
                                frame #3 {
                                n2129 = local read "H1 tt start hidden"() -> (w561:u32)
                                n2130 = local read "H1 tt end hidden"() -> (w562:u32)
                                n2131 = while {
                                tunnel: [w580] -> w576 mode=indexing
                                shift-right: [w581] -> _
                                shift-left: w557 -> [w583]
                                stop <- w578 stop-if-true
                                n2132 = Match Pattern(string=w583, regular expression=" ") -> (before substring=w580:string, after substring=w581:string, offset past match=w579:i32)  [unwired: 2 out]
                                n2133 = Less Than 0?(x=w579) -> (x < 0?=w578:bool)
                                }
                                n2134 = Subtract(x=w562, y=w561) -> (x-y=w560:u32)
                                n2135 = Divide(x=w560, y=u32 1000) -> (x/y=w558:dbl)
                                n2136 = local write "H1 measured Test Time"(w558) -> ()
                                n2137 = Array Size(array=w576) -> (size(s)=w573:i32)
                                n2138 = Divide(x=w573, y=3) -> (x/y=w575:dbl)
                                n2139 = To Unsigned Byte Integer(number=w575) -> (unsigned 8bit integer=w571:u8)
                                n2140 = local read "H1 SITES? response hid"() -> (w568:string)
                                n2141 = local read "H1 parallelism"() -> (w567:u32)
                                n2142 = Not Equal?(x=w567, y=w571) -> (x != y?=w572:bool)
                                n2143 = for {
                                N: w571 -> [_]
                                tunnel: w576 -> [w606]
